vi "Drag and Drop.vi"() -> ()   [LabVIEW 2011]
panel:
  out "To":i32(listbox)
  in  "From":i32(listbox)
  in  "stop":bool
  # "->"
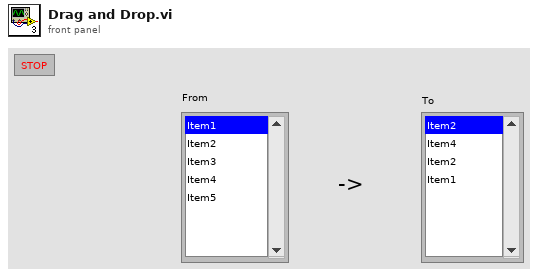
[diagram p1: front panel]
types:
  T1 = typedef "LVPoint32TypeDef.ctl" = cluster{"Horizontal":i32, "Vertical":i32}
  T2 = cluster{"data name":string, "drag data":variant}[]
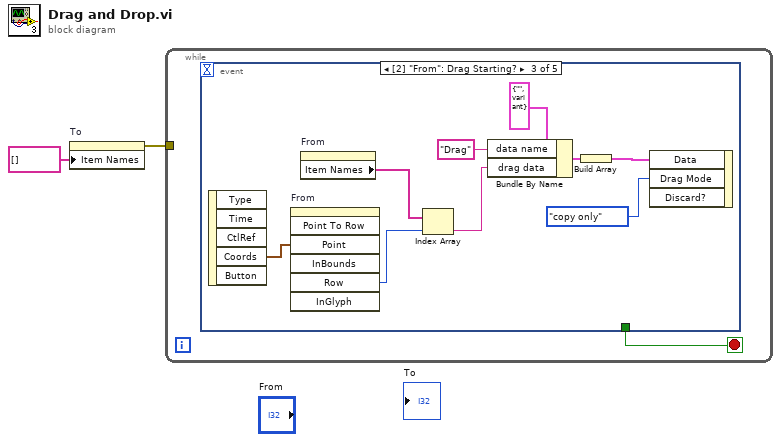
[diagram p0: block diagram]
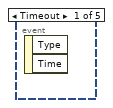
[diagram p2: hidden frame]
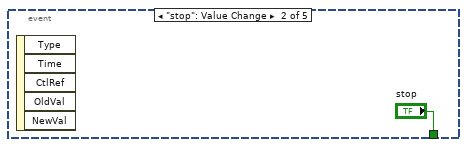
[diagram p3: hidden frame]
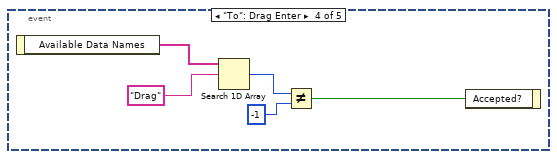
[diagram p4: hidden frame]
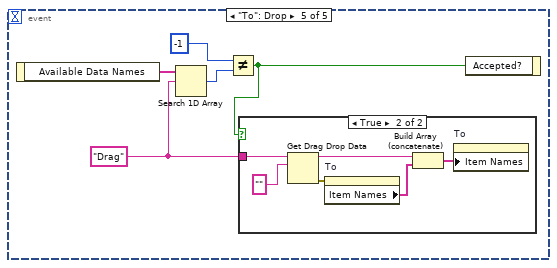
[diagram p5: hidden frame]
diagram:
  n1 = property on="To" class="LstBox (strict)"("Item Names"=string[] []) -> (error out=w2:errorcluster)  [unwired: 2 in, 1 out]
  n2 = while {
    tunnel: w2 -> [_]
    stop <- w3 stop-if-true
    n3 = event shown="[2] \"From\": Drag Starting?" {
      selector: _ -> [_ _ _ _ _]
      dyn-events: _ -> [_ _ _ _ _]
      timeout: _ -> [_ _ _ _ _]
      tunnel: [_ "stop" _ _ _] -> w3
      event Timeout {
        n4 = event-data() -> ()  [unwired: 1 in, 2 out]
      }
      event "stop": Value Change {
        n5 = event-data() -> ()  [unwired: 1 in, 5 out]
      }
      event "From": Drag Starting? {
        n6 = event-data() -> ("Coords"=w13:T1)  [unwired: 1 in, 4 out]
        n7 = invoke on="From" class="LstBox (strict)" method="Point To Row"("Point"=w13) -> ("Row"=w7:i32)  [unwired: 6 in, 6 out]
        n8 = property on="From" class="LstBox (strict)"() -> ("Item Names"=w8:string[])  [unwired: 2 in, 2 out]
        n9 = Index Array(array=w8, index=w7) -> (element=w6:string)
        n10 = Bundle By Name(cluster=cluster{"data name":string, "drag data":variant} {"data name"="", "drag data"=variant}, "data name"="Drag", "drag data"=w6) -> (w10:cluster{"data name":string, "drag data":variant})
        n11 = Build Array(w10) -> (w9:T2)
        n12 = event-data("Data"=w9, "Drag Mode"=enum32{"copy or move", "copy only", "move only"}."copy only") -> ()  [unwired: 2 in, 1 out]
      }
      event "To": Drag Enter {
        n13 = event-data() -> ("Available Data Names"=w18:string[])  [unwired: 1 in]
        n14 = Search 1D Array(1D array=w18, element="Drag") -> (index of element=w16:i32)  [unwired: 1 in]
        n15 = Not Equal?(x=w16, y=-1) -> (x != y?=w14:bool)
        n16 = event-data("Accepted?"=w14) -> ()  [unwired: 1 in, 1 out]
      }
      event "To": Drop {
        w22 = "Drag" ("data name")
        n17 = event-data() -> ("Available Data Names"=w23:string[])  [unwired: 1 in]
        n18 = Search 1D Array(1D array=w23, element=w22) -> (index of element=w20:i32)  [unwired: 1 in]
        n19 = Not Equal?(x=-1 ("y"), y=w20) -> (x != y?=w19:bool)
        n20 = case shown="True" w19 {
          tunnel: w22 -> [_ w24]
          frame False {
          }
          frame True {
            n21 = Get Drag Drop Data(8:"" ("type"), 9:w24) -> (0:w27:errorcluster, 3:w28:string)  [unwired: 1 in]
            n22 = property on="To" class="LstBox (strict)"(error in=w27) -> ("Item Names"=w26:string[])  [unwired: 1 in, 2 out]
            n23 = Build Array (concatenate)(w28, w26) -> (w25:string[])
            n24 = property on="To" class="LstBox (strict)"("Item Names"=w25) -> ()  [unwired: 2 in, 2 out]
          }
        }
        n25 = event-data("Accepted?"=w19) -> ()  [unwired: 1 in, 1 out]
      }
    }
  }
